vi "Untitled 1.vi"() -> ()   [LabVIEW 2015]
uses:
  MathLibrary.dll
panel:
  out "Numeric 3":dbl
  in  "Numeric 2":dbl
  in  "Numeric":dbl
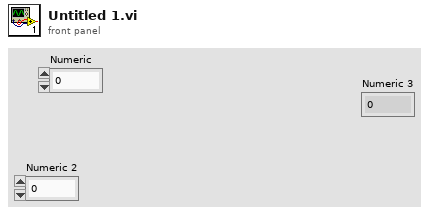
[diagram p1: front panel]
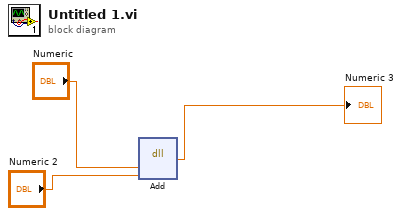
[diagram p0: block diagram]
diagram:
  n1 = dll-call lib="D:/PROIECT DRONA/MathLibrary.dll" fn="Add"("arg1"="Numeric", "arg2"="Numeric 2") -> ("return type"=→"Numeric 3":dbl)  [unwired: 5 in, 2 out]
